vi "Read Format String.vi"(8 "error in (no error)":errorcluster, 11 "NT Scalar (Numeric) in":refnum<class "NT Scalar (Numeric).lvclass">) -> (0 "error out":errorcluster, 2 "format string":string, 3 "NT Scalar (Numeric) out":refnum<class "NT Scalar (Numeric).lvclass">)   [LabVIEW 2020, in "PV Access.lvlib" / "PV Data.lvlib" / "NT Scalar (Numeric).lvclass"]
uses:
  NT Scalar (Numeric).lvclass
  NT Scalar (Numeric).lvclass/NT Scalar (Numeric).ctl
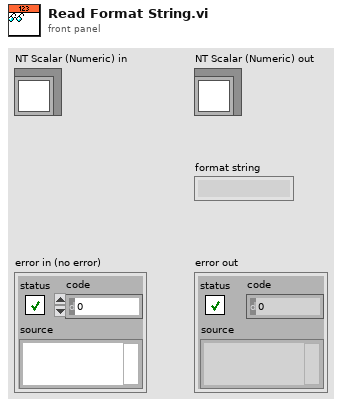
[diagram p1: front panel]
types:
  T1 = typedef "PV Access.lvlib/PV Data.lvlib/Display Form.ctl" = enum32{"Default", "String", "Binary", "Decimal", "Hex", "Exponential", "Engineering"}
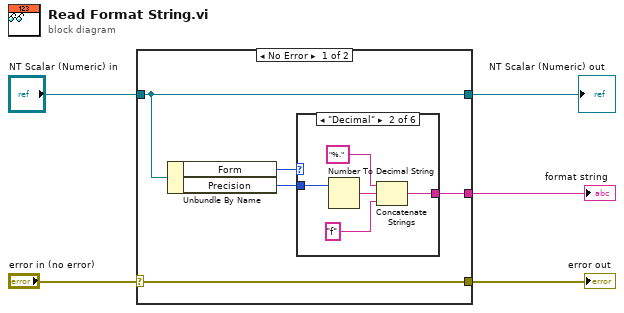
[diagram p0: block diagram]
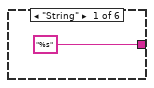
[diagram p2: hidden frame]
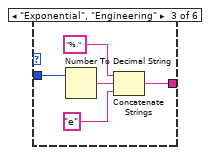
[diagram p3: hidden frame]
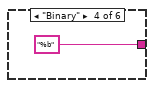
[diagram p4: hidden frame]
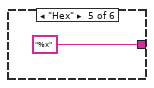
[diagram p5: hidden frame]
diagram:
  n1 = case shown="No Error" "error in (no error)" {
    selector: "error in (no error)" -> [w10 w24]
    tunnel: [w10 w24] -> w4
    tunnel: [w9 w25] -> w2
    tunnel: "NT Scalar (Numeric) in" -> [w9 w25]
    tunnel: [w8 _] -> w1
    frame No Error {
      n2 = Unbundle By Name(w9) -> ("Form"=w7:T1, "Precision"=w6:i32)
      n3 = case shown="\"Decimal\"" w7 {
        tunnel: w6 -> [_ w16 w21 _ _ _]
        tunnel: ["%s" w15 w19 "%b" "%x" _] -> w8
        frame "String" {
        }
        frame "Decimal" {
          n4 = Number To Decimal String(number=w16) -> (decimal integer string=w14:string)  [unwired: 1 in]
          n5 = Concatenate Strings("%.", w14, "f") -> (w15:string)
        }
        frame "Exponential", "Engineering" {
          n6 = Number To Decimal String(number=w21) -> (decimal integer string=w18:string)  [unwired: 1 in]
          n7 = Concatenate Strings("%.", w18, "e") -> (w19:string)
        }
        frame "Binary" {
        }
        frame "Hex" {
        }
        frame Default {
        }
      }
    }
    frame Error {
    }
  }
  "error out" <- w4
  "NT Scalar (Numeric) out" <- w2
  "format string" <- w1
